vi "周期测量_高频.vi"() -> ()   [LabVIEW 2013]
doc: "This example demonstrates how to count the pulse's edges."
uses:
  <userlib>/ArtDAQ/_SubVI/ArtDAQ_CreateCIPeriodChan.vi
  <userlib>/ArtDAQ/_SubVI/ArtDAQ_CfgSampClkTiming.vi
  <userlib>/ArtDAQ/_SubVI/ArtDAQ_Read Counter DBL NSamp.vi
panel:
  in  "开始边沿":i32(ring)=10280 items=["上升"=10280, "下降"=10171]
  in  "测量时间":dbl=0.01 format="%#_13g"
  in  "每通道点数":i32=100
  in  "采样速率":dbl=10000.0 format="%#_13g"
  in  "有效边沿":i32(ring)=10280 items=["上升"=10280, "下降"=10171]
  in  "时钟源":string="/Dev1/PFI1"
  out "数据":dbl[](array[numeric]) format="%_6g"
  in  "计数器":string="Dev1/ctr0"
  in  "最小值":dbl=1e-06 format="%0.6f"
  in  "最大值":dbl=10.0 format="%0.6f"
  in  "Stop":bool
  out "错误输出":errorcluster
  # "定时"
  # "通道属性"
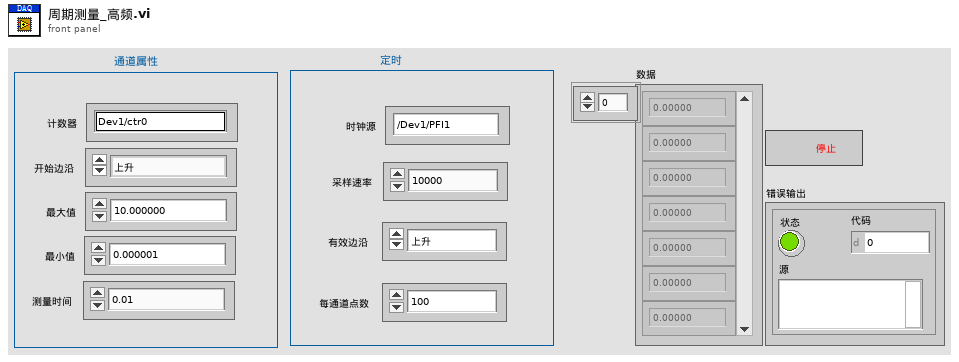
[diagram p1: front panel]
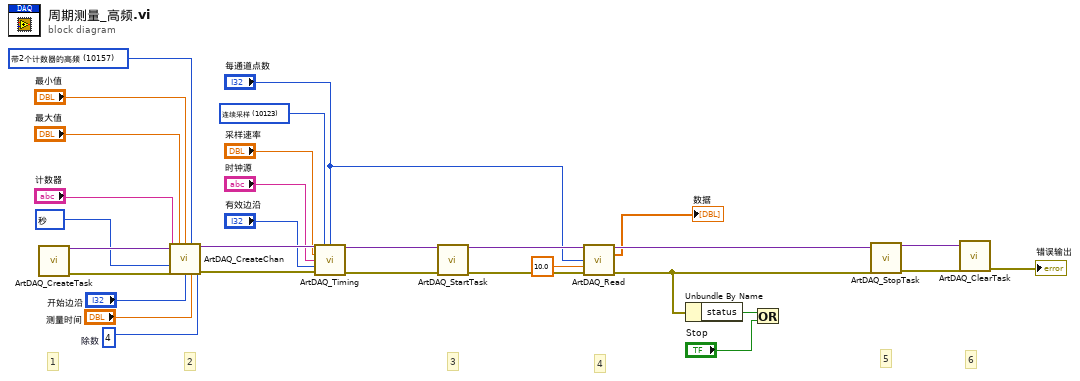
[diagram p0: block diagram]
diagram:
  w10 = u32 4  # 除数
  w6 = 10364 items=["秒"=10364, "时钟滴答"=10304, "来自自定义换算"=10065] ("单位")
  w13 = 10157 items=["带1个计数器的低频"=10105, "带2个计数器的高频"=10157, "带2个计数器的大范围"=10205] ("测试方法")
  w14 = 10123 items=["有限点采样"=10178, "连续采样"=10123] ("采样模式")
  # "4"
  # "6"
  # "5"
  # "3"
  # "2"
  # "1"
  n1 = call <userlib>:"ArtDAQ_CreateTask.vi"() -> ("任务句柄"=w30:variant, "错误输出"=w29:errorcluster)  [unwired: 14 in]
  n2 = call-poly <userlib>:"ArtDAQ_CreateChan.vi"("任务句柄"=w30, "最大值"="最大值", "最小值"="最小值", "测量方法"=w13, "计数器"="计数器", "除数"=w10, "单位"=w6, "错误输入"=w29, "开始边沿"="开始边沿", "测量时间"="测量时间") -> ("任务句柄"=w18:variant, "错误输出"=w15:errorcluster)  [unwired: 4 in]
  n3 = call-poly <userlib>:"ArtDAQ_Timing.vi"("任务句柄"=w18, "采样模式"=w14, "每通道采样数"="每通道点数", "采样率"="采样速率", "源"="时钟源", "有效边沿"="有效边沿", "错误输入"=w15) -> ("任务句柄"=w17:variant, "错误输出"=w16:errorcluster)  [unwired: 7 in]
  n4 = call <userlib>:"ArtDAQ_StartTask.vi"("任务句柄"=w17, "错误输入"=w16) -> ("任务句柄"=w22:variant, "错误输出"=w21:errorcluster)  [unwired: 12 in]
  n5 = call-poly <userlib>:"ArtDAQ_Read.vi"("任务句柄"=w22, "每通道采样数"="每通道点数", "超时s"=10.0 ("Timeout"), "错误输入"=w21) -> ("任务句柄"=w27:variant, "数据"=→"数据":dbl[], "错误输出"=w25:errorcluster)  [unwired: 8 in, 1 out]
  n6 = Unbundle By Name(w25) -> ("status"=w4:bool)
  n7 = Or(x=w4, y="Stop") -> ()  [unwired: 1 out]
  n8 = call <userlib>:"ArtDAQ_StopTask.vi"("任务句柄"=w27, "错误输入"=w25) -> ("任务句柄"=w26:variant, "错误输出"=w24:errorcluster)  [unwired: 12 in]
  n9 = call <userlib>:"ArtDAQ_ClearTask.vi"("任务句柄"=w26, "错误输入"=w24) -> ("错误输出"=→"错误输出":errorcluster)  [unwired: 13 in]
